vi "Servo_Write.vi"(2 "error in (no error)":errorcluster, 3 "Servo Index":u8, 4 "Servo Control":dbl(slide) scale=0.0..180.0, 5 "VISA resource name":refnum<visa-resource-name>) -> (0 "error out":errorcluster, 1 "VISA resource name out":refnum<visa-resource-name>)   [LabVIEW 2023]
doc: "Takes a Target Value in Servo Control from 0 to 180 (degrees) and sends the according pulse length and servo index (1 to 4) to the controller."
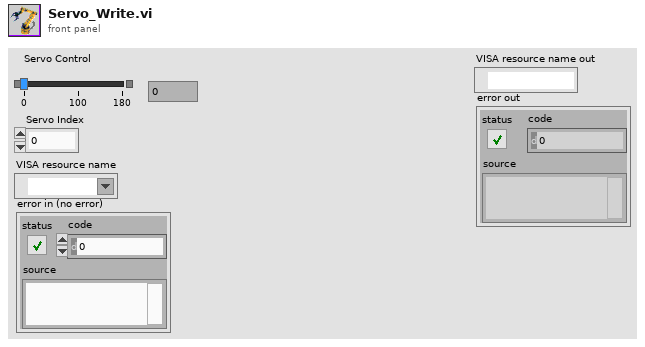
[diagram p1: front panel]
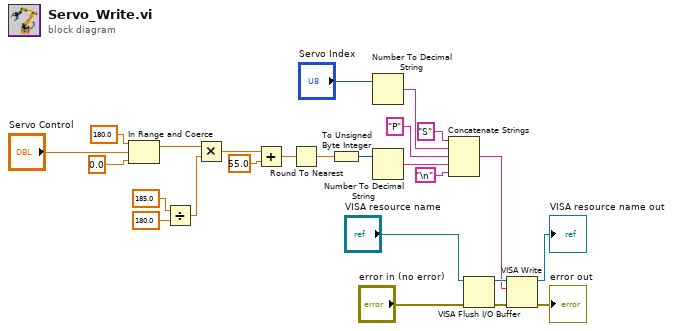
[diagram p0: block diagram]
diagram:
  n1 = In Range and Coerce(upper limit=180.0, x="Servo Control", lower limit=0.0) -> (coerced(x)=w11:dbl)  [unwired: 1 out]
  n2 = Divide(x=185.0, y=180.0) -> (x/y=w17:dbl)
  n3 = Multiply(x=w11, y=w17) -> (x*y=w9:dbl)
  n4 = Add(x=w9, y=55.0) -> (x+y=w10:dbl)
  n5 = Round To Nearest(number=w10) -> (nearest integer value=w16:dbl)
  n6 = To Unsigned Byte Integer(number=w16) -> (unsigned 8bit integer=w15:u8)
  n7 = Number To Decimal String(number="Servo Index") -> (decimal integer string=w20:string)  [unwired: 1 in]
  n8 = Number To Decimal String(number=w15) -> (decimal integer string=w24:string)  [unwired: 1 in]
  n9 = Concatenate Strings("S" ("string"), w20, "P" ("string"), w24, "\n") -> (w1:string)
  n10 = VISA Flush I/O Buffer(VISA resource name="VISA resource name", error in (no error)="error in (no error)") -> (VISA resource name out=w6:refnum<visa-resource-name>, error out=w7:errorcluster)  [unwired: 1 in]
  n11 = VISA Write(VISA resource name=w6, write buffer=w1, error in (no error)=w7) -> (VISA resource name out=→"VISA resource name out":refnum<visa-resource-name>, error out=→"error out":errorcluster)  [unwired: 1 out]
